vi "write_attributes.vi"(8 "error in (no error)":errorcluster, 10 "attributes":T1, 11 "MiniBatchKMeans in":refnum<class "MiniBatchKMeans.lvclass">) -> (0 "error out":errorcluster, 3 "MiniBatchKMeans out":refnum<class "MiniBatchKMeans.lvclass">)   [LabVIEW 2020, in "MiniBatchKMeans.lvclass"]
uses:
  MiniBatchKMeans.lvclass
  Controls/mini_batch_kmeans_attributes.ctl
  MiniBatchKMeans.lvclass/MiniBatchKMeans.ctl
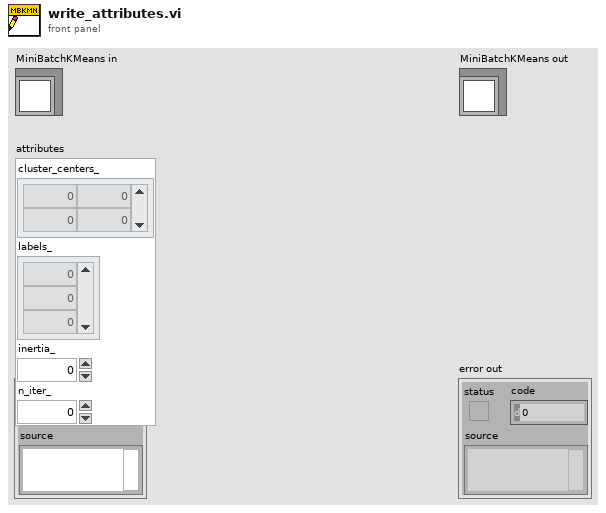
[diagram p1: front panel]
types:
  T1 = typedef "mini_batch_kmeans_attributes.ctl" = cluster{"cluster_centers_":dbl[][], "labels_":dbl[], "inertia_":dbl, "n_iter_":dbl}
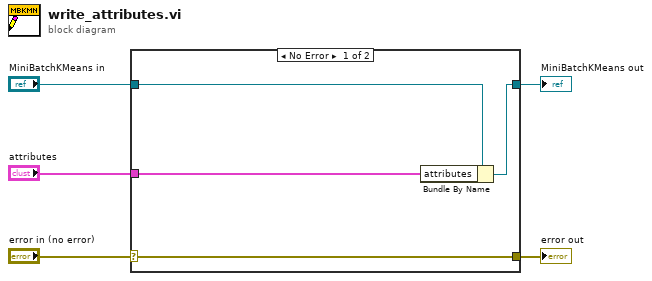
[diagram p0: block diagram]
diagram:
  n1 = case shown="No Error" "error in (no error)" {
    selector: "error in (no error)" -> [w9 w10]
    tunnel: [w9 w10] -> w4
    tunnel: [w7 w11] -> w2
    tunnel: "MiniBatchKMeans in" -> [w8 w11]
    tunnel: "attributes" -> [w6 _]
    frame No Error {
      n2 = Bundle By Name(cluster=w8, "attributes"=w6) -> (w7:refnum<class "MiniBatchKMeans.lvclass">)
    }
    frame Error {
    }
  }
  "error out" <- w4
  "MiniBatchKMeans out" <- w2
